vi "Create Footer Text.vi"(0 "Module Init Timestamp":timestamp, 1 "Module Close Timestamp":timestamp, 2 "Error_Log_Setting":T1, 3 "Total no. of errors reported":i32, 4 "Total no. of errors handled":i32) -> (5 "Footer to be written to error log file":string, 6 "Number of characters":i32)   [LabVIEW 2023, in "Error Manager.lvlib" / "Error Log.lvclass"]
uses:
  Error Log.lvclass
  Error Log.lvclass/Error Log.ctl
  Error Manager.lvlib
  Settings/Error_Log_Setting (enum).ctl
  Settings/Settings.lvclass
panel:
  # "Input\nInputs to the VI"
  # "Development\nControls or indicators that are useful for development or testing, but which are not outputs of the VI."
  # "Output\nOutputs of the VI"
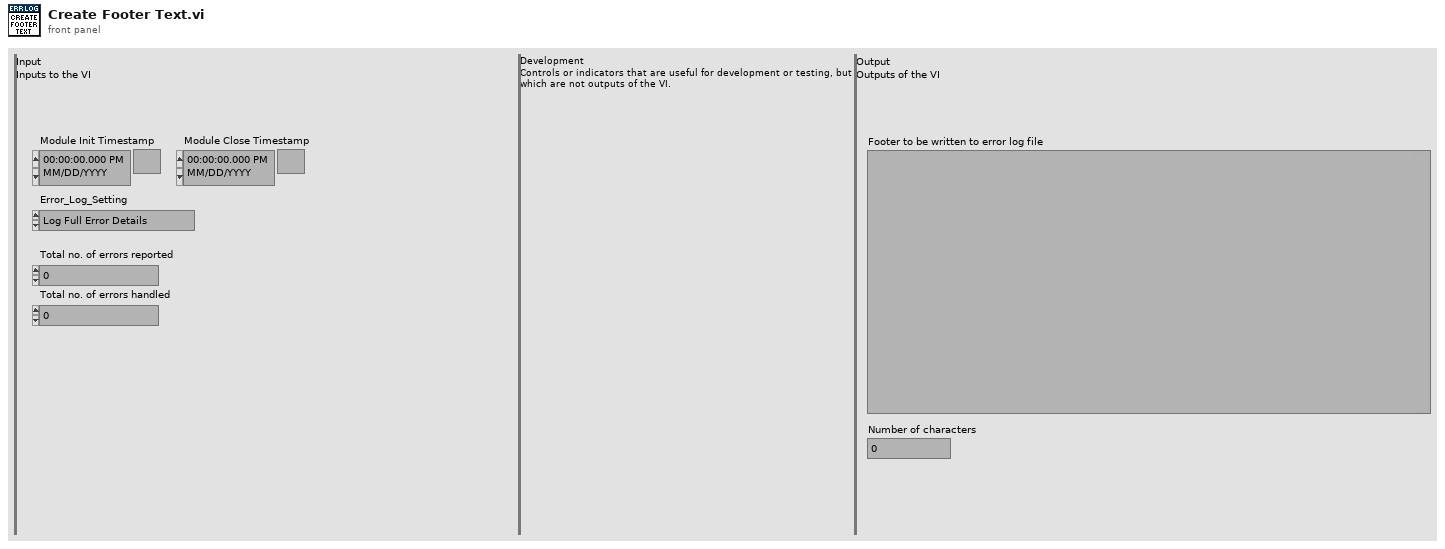
[diagram p1: front panel]
types:
  T1 = typedef "Error Manager.lvlib/Settings.lvclass/Error_Log_Setting (enum).ctl" = enum16{"Log Full Error Details", "Log Error Codes Only", "Do Not Log"}
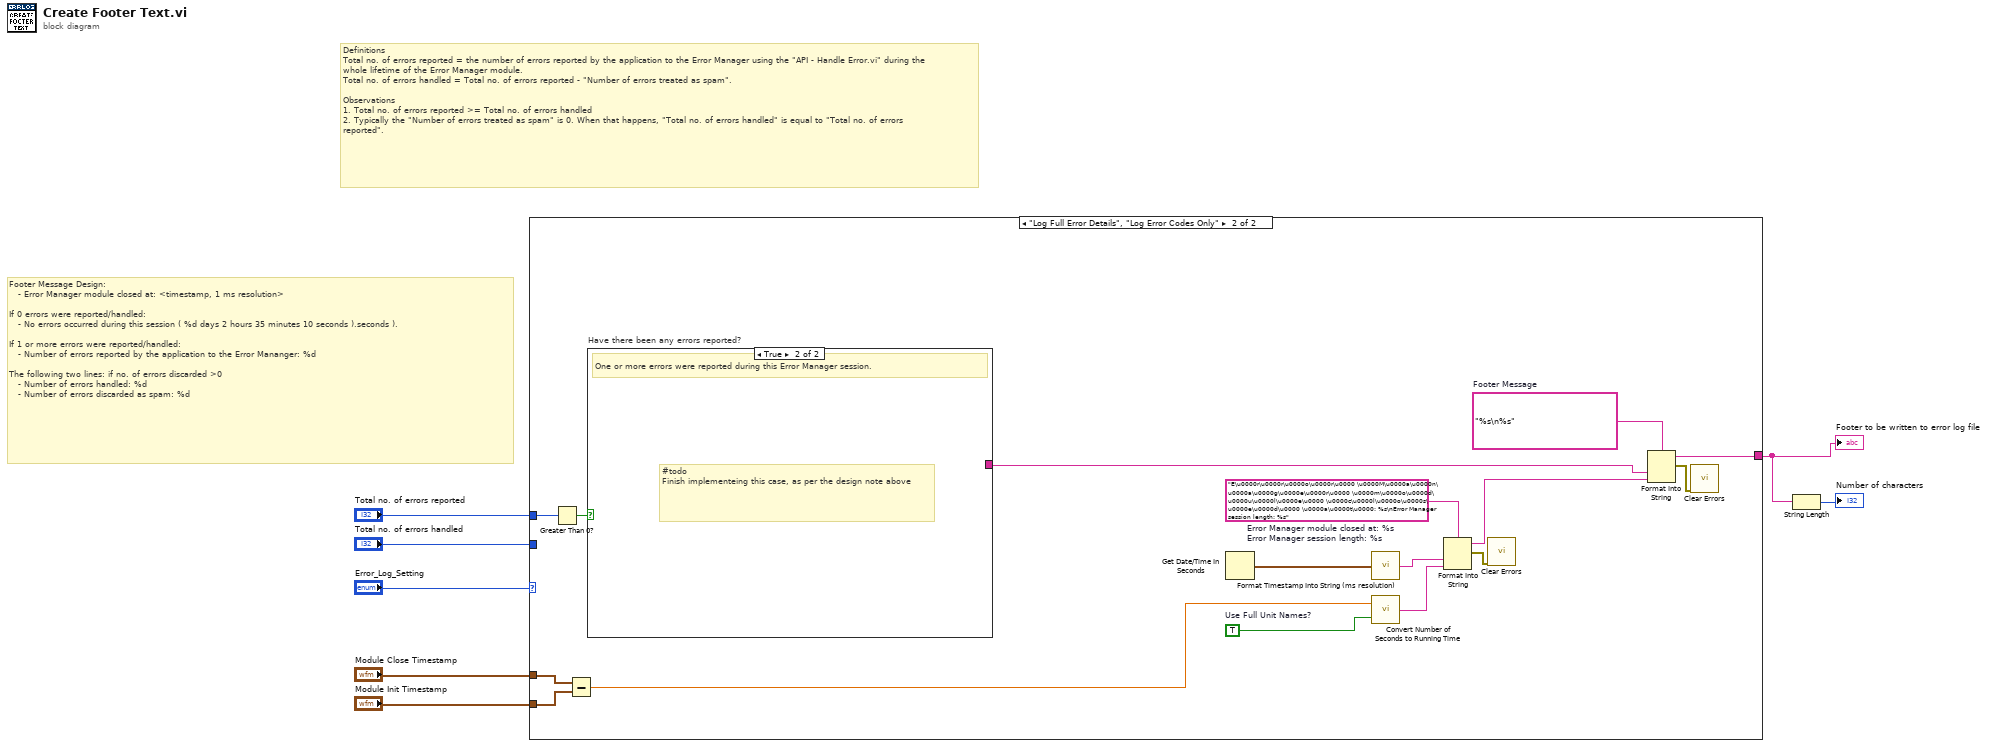
[diagram p0: block diagram]
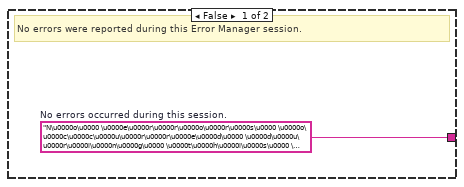
[diagram p3: hidden frame]
diagram:
  # "Definitions\nTotal no. of errors reported = the number of errors reported by the application to the Error Manager using the \"API - Handle Error.vi\" during the whole lifetime of the Error Manager module.\nTotal no. of errors handled = Total no. of errors reported - \"Number of errors treated as spam\".\n\nObservations\n1. Total no. of errors reported >= Total no. of errors handled\n2. Typically the \"Number of errors treated as spam\" is 0. When that happens, \"Total no. of errors handled\" is equal to \"Total no. of errors reported\"."
  # "Footer Message Design:\n   - Error Manager module closed at: <timestamp, 1 ms resolution>\n\nIf 0 errors were reported/handled:\n   - No errors occurred during this session ( %d days 2 hours 35 minutes 10 seconds ).seconds ).\n\nIf 1 or more errors were reported/handled:\n   - Number of errors reported by the application to the Error Mananger: %d\n\nThe following two lines: if no. of errors discarded >0\n   - Number of errors handled: %d\n   - Number of errors discarded as spam: %d"
  n1 = case shown="\"Log Full Error Details\", \"Log Error Codes Only\"" "Error_Log_Setting" {
    tunnel: [_ w18] -> w7
    tunnel: "Total no. of errors reported" -> [_ w16]
    tunnel: "Total no. of errors handled" -> [_ _]
    tunnel: "Module Close Timestamp" -> [_ w13]
    tunnel: "Module Init Timestamp" -> [_ w12]
    frame "Do Not Log" {
    }
    frame "Log Full Error Details", "Log Error Codes Only" {
      w10 = TRUE  # Use Full Unit Names?
      w20 = "%s\n%s"  # Footer Message
      w23 = "E\u0000r\u0000r\u0000o\u0000r\u0000 \u0000M\u0000a\u0000n\u0000a\u0000g\u0000e\u0000r\u0000 \u0000m\u0000o\u0000d\u0000u\u0000l\u0000e\u0000 \u0000c\u0000l\u0000o\u0000s\u0000e\u0000d\u0000 \u0000a\u0000t\u0000: %s\nError Manager session length: %s"  # Error Manager module closed at: %s Error Manager session length: %s
      n2 = Greater Than 0?(x=w16) -> (x > 0?=w15:bool)
      n3 = Subtract(x=w13, y=w12) -> (x-y=w11:dbl)
      n4 = case "Have there been any errors reported?" shown="True" w15 {
        tunnel: [w24 _] -> w14
        frame False {
          w24 = "N\u0000o\u0000 \u0000e\u0000r\u0000r\u0000o\u0000r\u0000s\u0000 \u0000o\u0000c\u0000c\u0000u\u0000r\u0000r\u0000e\u0000d\u0000 \u0000d\u0000u\u0000r\u0000i\u0000n\u0000g\u0000 \u0000t\u0000h\u0000i\u0000s\u0000 \u0000s\u0000e\u0000s\u0000s\u0000i\u0000o\u0000n\u0000."  # No errors occurred during this session.
          # "No errors were reported during this Error Manager session."
        }
        frame True {
          # "#todo\nFinish implementeing this case, as per the design note above"
          # "One or more errors were reported during this Error Manager session."
        }
      }
      n5 = Get Date/Time In Seconds() -> (seconds since 1Jan1904=w17:timestamp)
      n6 = call "Format Timestamp Into String (ms resolution).vi"("Timestamp"=w17) -> ("Timestamp String (ms resolution)"=w22:string)
      n7 = call "Convert Number of Seconds to Running Time.vi"("Use Full Unit Names? (F)"=w10, "Number of seconds elapsed"=w11) -> ("Running Time String"=w9:string)
      n8 = Format Into String(format string=w23, w22, w9) -> (resulting string=w8:string, error out=w21:errorcluster)  [unwired: 2 in]
      n9 = call <vilib>:"Clear Errors.vi"("error in (no error)"=w21) -> ()  [unwired: 5 in, 2 out]
      n10 = Format Into String(format string=w20, w14, w8) -> (resulting string=w18:string, error out=w19:errorcluster)  [unwired: 2 in]
      n11 = call <vilib>:"Clear Errors.vi"("error in (no error)"=w19) -> ()  [unwired: 5 in, 2 out]
    }
  }
  "Footer to be written to error log file" <- w7
  n12 = String Length(string=w7) -> (length=→"Number of characters":i32)
